vi "Get Config.vi"(8 "error in (no error)":errorcluster, 11 "GroupAbstract in":refnum<class "GroupAbstract.lvclass">) -> (0 "error out":errorcluster, 2 "Config":refnum<class "Group Config.lvclass">, 3 "GroupAbstract out":refnum<class "GroupAbstract.lvclass">)   [LabVIEW 2020, in "Vecto.lvlib" / "GroupAbstract.lvclass"]
uses:
  GroupAbstract.lvclass
  Group Config/Group Config.lvclass
  GroupAbstract.lvclass/GroupAbstract.ctl
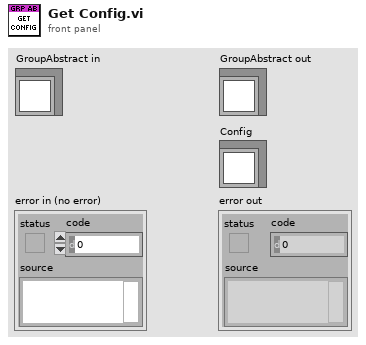
[diagram p1: front panel]
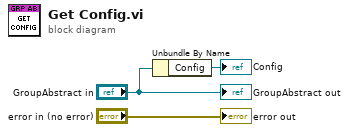
[diagram p0: block diagram]
diagram:
  n1 = Unbundle By Name("GroupAbstract in") -> ("Config"=→"Config":refnum<class "Group Config.lvclass">)
  "error out" <- "error in (no error)"
  "GroupAbstract out" <- "GroupAbstract in"
